vi "Is Command within a Preset.vi"(8 "error in (no error)":errorcluster, 10 "Index of command":i32, 11 "Macro Array IN":string[](array[string])) -> (0 "error out":errorcluster, 2 "Index of Preset.Start":i32, 3 "Part of a Macro?":bool)   [LabVIEW 2012]
doc: "SciScan 1.2 160622"
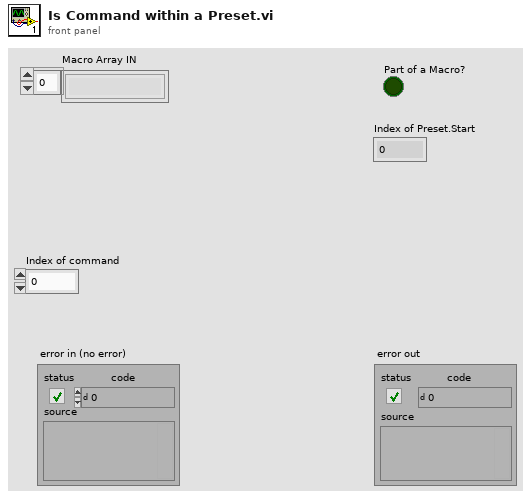
[diagram p1: front panel]
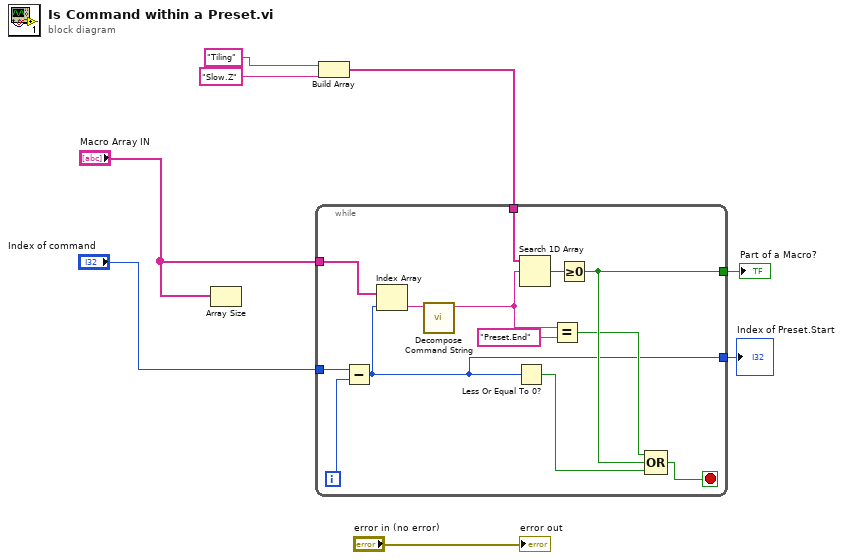
[diagram p0: block diagram]
diagram:
  n1 = Array Size(array="Macro Array IN") -> ()  [unwired: 1 out]
  n2 = Build Array("Tiling" ("element"), "Slow.Z" ("element")) -> (w5:string[])
  n3 = while {
    tunnel: "Index of command" -> [w21]
    tunnel: w5 -> [w18]
    tunnel: "Macro Array IN" -> [w16]
    tunnel: [w14] -> w3
    tunnel: [w9] -> w1
    i -> [w20]
    stop <- w13 stop-if-true
    n4 = Subtract(x=w21, y=w20) -> (x-y=w9:i32)
    n5 = Index Array(array=w16, index=w9) -> (element=w17:string)
    n6 = call "Decompose Command String.vi"("Command IN"=w17) -> ("Action"=w12:string)  [unwired: 7 in, 3 out]
    n7 = Less Or Equal To 0?(x=w9) -> (x <= 0?=w19:bool)
    n8 = Search 1D Array(1D array=w18, element=w12) -> (index of element=w15:i32)  [unwired: 1 in]
    n9 = Equal?(x=w12, y="Preset.End") -> (x = y?=w10:bool)
    n10 = Greater Or Equal To 0?(x=w15) -> (x >= 0?=w14:bool)
    n11 = Compound Arithmetic op=OR(w10, w14, w19) -> (w13:bool)
  }
  "Part of a Macro?" <- w3
  "Index of Preset.Start" <- w1
  "error out" <- "error in (no error)"
